vi "Init.vi"(8 "Error In":errorcluster, 9 "Stop Button Refnum":refnum<vi>, 10 "Data Refnum":refnum<vi>, 11 "Card # Refnum":refnum<vi>) -> (0 "error out":errorcluster)   [LabVIEW 2013, in "Display Panel Non-Actor Class.lvlib" / "Display Panel Non-Actor Class.lvclass"]
uses:
  Display Panel Non-Actor Class.lvclass
  Controls/Numeric Indicator.ctl
panel:
  in  "Display Panel Non-Actor Class.lvlib:Display Panel Non-Actor Class.lvclass":refnum<class "Display Panel Non-Actor Class.lvclass">
  out "Display Panel Non-Actor Class out":refnum<class "Display Panel Non-Actor Class.lvclass">
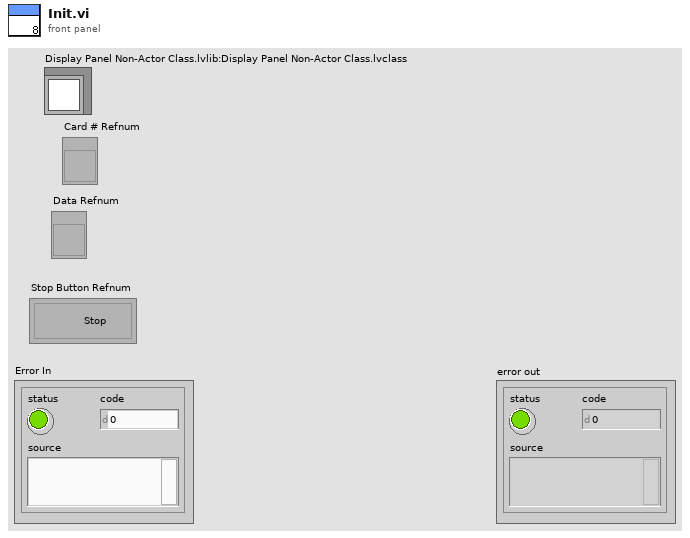
[diagram p1: front panel]
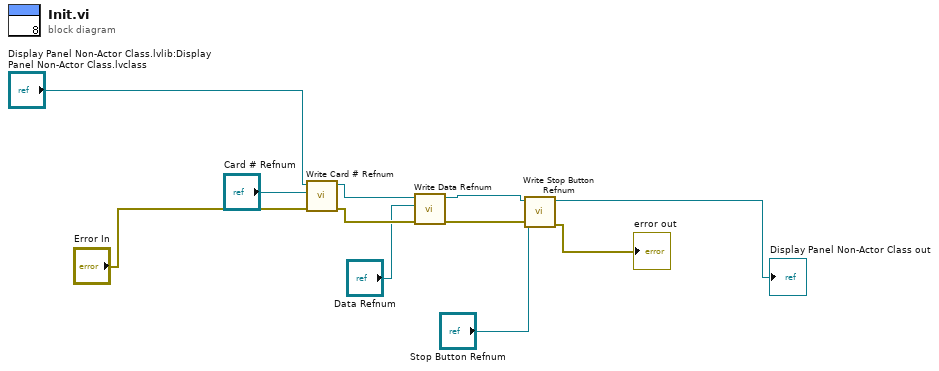
[diagram p0: block diagram]
diagram:
  n1 = call-dynamic "Write Card # Refnum.vi"("error in (no error)"="Error In", "Card # Refnum"="Card # Refnum", "Display Panel Non-Actor Class in"="Display Panel Non-Actor Class.lvlib:Display Panel Non-Actor Class.lvclass") -> ("error out"=w7:errorcluster, "Display Panel Non-Actor Class out"=w9:refnum<class "Display Panel Non-Actor Class.lvclass">)  [unwired: 7 in]
  n2 = call-dynamic "Write Data Refnum.vi"("error in (no error)"=w7, "Data Refnum"="Data Refnum", "Display Panel Non-Actor Class in"=w9) -> ("error out"=w6:errorcluster, "Display Panel Non-Actor Class out"=w8:refnum<class "Display Panel Non-Actor Class.lvclass">)  [unwired: 7 in]
  n3 = call-dynamic "Write Stop Button Refnum.vi"("error in (no error)"=w6, "Stop Button Refnum"="Stop Button Refnum", "Display Panel Non-Actor Class in"=w8) -> ("error out"=→"error out":errorcluster, "Display Panel Non-Actor Class out"=→"Display Panel Non-Actor Class out":refnum<class "Display Panel Non-Actor Class.lvclass">)  [unwired: 7 in]
